vi "movimentacao_cin_inv_bezier.vi"() -> ()   [LabVIEW 2017]
doc: "The myRIO Project template acquires acceleration data from the onboard accelerometer and displays the changes of acceleration values in a waveform chart."
uses:
  <vilib>/Analysis/Matrix/Datatypes/RealMatrix.ctl
  <vilib>/myRIO/Instrument Drivers/Onboard IO/PWM/typedefs/PWM Reference.ctl
  <vilib>/myRIO/Common/Instrument Driver Framework/Utilities/typedefs/myRIO Generic Hardware Reference.ctl
  <vilib>/myRIO/Common/Instrument Driver Framework/Utilities/typedefs/Hardware Version Enum.ctl
  <vilib>/myRIO/Common/Instrument Driver Framework/Utilities/typedefs/myRIO v1.0 Reference.ctl
  <vilib>/myRIO/Common/Instrument Driver Framework/Utilities/typedefs/Generic FPGA Reference.ctl
  <vilib>/myRIO/Common/Instrument Driver Framework/myRIO v1.0/PWM/typedefs/PWM Channels Enum.ctl
  <vilib>/myRIO/Instrument Drivers/Onboard IO/PWM/typedefs/PWM Configuration.ctl
  <vilib>/userdefined/High Color/nirio_resource_hc.ctl
  <vilib>/myRIO/Common/Instrument Driver Framework/myRIO v1.0/PWM/vis/myRIO v1.1 Open PWM.vi
  <vilib>/myRIO/Common/Instrument Driver Framework/Utilities/vis/Validate Channels.vi
  <vilib>/myRIO/Common/Instrument Driver Framework/myRIO v1.0/PWM/vis/myRIO v1.0 Reserve PWM.vi
  <vilib>/myRIO/Instrument Drivers/Onboard IO/PWM/vis/Set Duty Cycle and Frequency.vi
  <vilib>/myRIO/Common/Instrument Driver Framework/myRIO v1.0/PWM/vis/myRIO v1.0 Close PWM.vi
  <vilib>/myRIO/Common/Instrument Driver Framework/myRIO v1.0/PWM/vis/myRIO v1.0 Build MUX Configuration PWM.vi
  <vilib>/myRIO/Common/Instrument Driver Framework/myRIO v1.0/Resource Manager/vis/myRIO v1.0 Reserve Channel List.vi
  <vilib>/myRIO/Common/Instrument Driver Framework/myRIO v1.0/PWM/vis/myRIO v1.0 Unreserve PWM.vi
  <vilib>/myRIO/Common/Instrument Driver Framework/myRIO v1.0/Resource Manager/vis/myRIO v1.0 Create Configuration List.vi
  <vilib>/myRIO/Common/Instrument Driver Framework/myRIO v1.0/Resource Manager/vis/myRIO v1.0 Reserve Channel.vi
  <vilib>/myRIO/Common/Instrument Driver Framework/myRIO v1.0/Resource Manager/vis/myRIO v1.0 Unreserve Channel.vi
  <vilib>/myRIO/Common/Instrument Driver Framework/myRIO v1.0/Resource Manager/vis/myRIO v1.0 Unreserve Channel List.vi
  <vilib>/myRIO/Common/Instrument Driver Framework/myRIO v1.0/Resource Manager/vis/myRIO v1.0 Build Mutex Name.vi
  <vilib>/Utility/VariantDataType/GetNumericInfo.vi
  <vilib>/Utility/error.llb/Error Cluster From Error Code.vi
  <vilib>/myRIO/Common/Instrument Driver Framework/myRIO v1.0/myRIO v1.1 Open.vi
  <vilib>/myRIO/Common/Instrument Driver Framework/Utilities/vis/IO Manager.vi
  <vilib>/myRIO/Common/Instrument Driver Framework/Utilities/vis/Configuration Manager.vi
  <vilib>/myRIO/Common/Instrument Driver Framework/myRIO v1.0/Resource Manager/vis/myRIO v1.0 Configure IO.vi
  <vilib>/myRIO/Common/Instrument Driver Framework/myRIO v1.0/myRIO v1.0 Close.vi
  <vilib>/myRIO/Common/Instrument Driver Framework/myRIO v1.0/PWM/vis/myRIO v1.0 Write PWM.vi
  <vilib>/myRIO/Common/Instrument Driver Framework/myRIO v1.0/PWM/vis/myRIO v1.0 Shutdown PWM.vi
  <vilib>/myRIO/Instrument Drivers/Onboard IO/PWM/vis/myRIO PWM Open.xnode
  <vilib>/myRIO/Instrument Drivers/Onboard IO/PWM/PWM.lvlib
  <vilib>/Analysis/Matrix/NI_Matrix.lvlib
panel:
  in  "String 3":string="(151,57;2,89;11,57);(245,79;-185,54;30);(126,28;-267,6;41,68);(43,16; -253,15;220,9);(-167,79;-132,49;100)"
  out "x .and. y?":bool
  in  "OK Button":bool
  out "subarray":dbl[](array[numeric])
  in  "String 2":string="(151,57;2,89;11,57);(245,79;-185,54;30);(126,28;-267,6;41,68);(43,16; -253,15;220,9);(-167,79;-132,49;100)"
  out "output array":T1
  out "appended array 2":dbl[](array[numeric])
  out "logical AND":bool
  out "x = y?":bool[](array[boolean])
  out "POS_E_ORIEN_HOME":dbl[](array[numeric])
  out "ANG_POSI_E_ORIEN_HOME":dbl[](array[numeric])
  out "CURRENT POSITIONS OF THE MOTORS":dbl[](array[numeric])
  in  "angulo_garra":dbl(knob) scale=-180.0..180.0
  in  "Duty Cycle Abert":dbl=0.04 format="%#_13g"
  out "Actuator 2":bool
  in  "Actuator":bool
  in  "Conveyor speed (mm/s)":dbl(slide)=200.0 step=1.0 scale=0.0..350.0
  out "indexador":i32
  out "Objeto detectado":bool
  out "Manipulando":bool
  out "Está em Home":bool
  out "Posicao_desejada":bool
  in  "Home":bool
  in  "error in (no error)":errorcluster
  in  "PARAR":bool
  in  "POSITION VECTOR":dbl[](array[numeric])
  # "ROTINA DE CONTROLE DO PROTÓTIPO DE FMS"
  # "COMANDO DE POSIÇÃO\nATUAL DOS MOTORES"
  # "OPERATION STATUS"
  # "ÂNGULOS DE JUNTAS"
  # "THETA 1"
  # "MOTOR 1"
  # "HOME"
  # "THETA 2"
  # "MOTOR 2"
  # "DESIRED POSITION"
  # "THETA 3"
  # "MOTOR 3"
  # "OBJECT DETECTED"
  # "THETA 4"
  # "MOTOR 4"
  # "MANIPULATING"
  # "THETA 5"
  # "MOTOR 5"
  # "ACTUATOR"
  # "MOTOR 6"
  # "VELOCIDADE DA ESTEIRA (mm/s)"
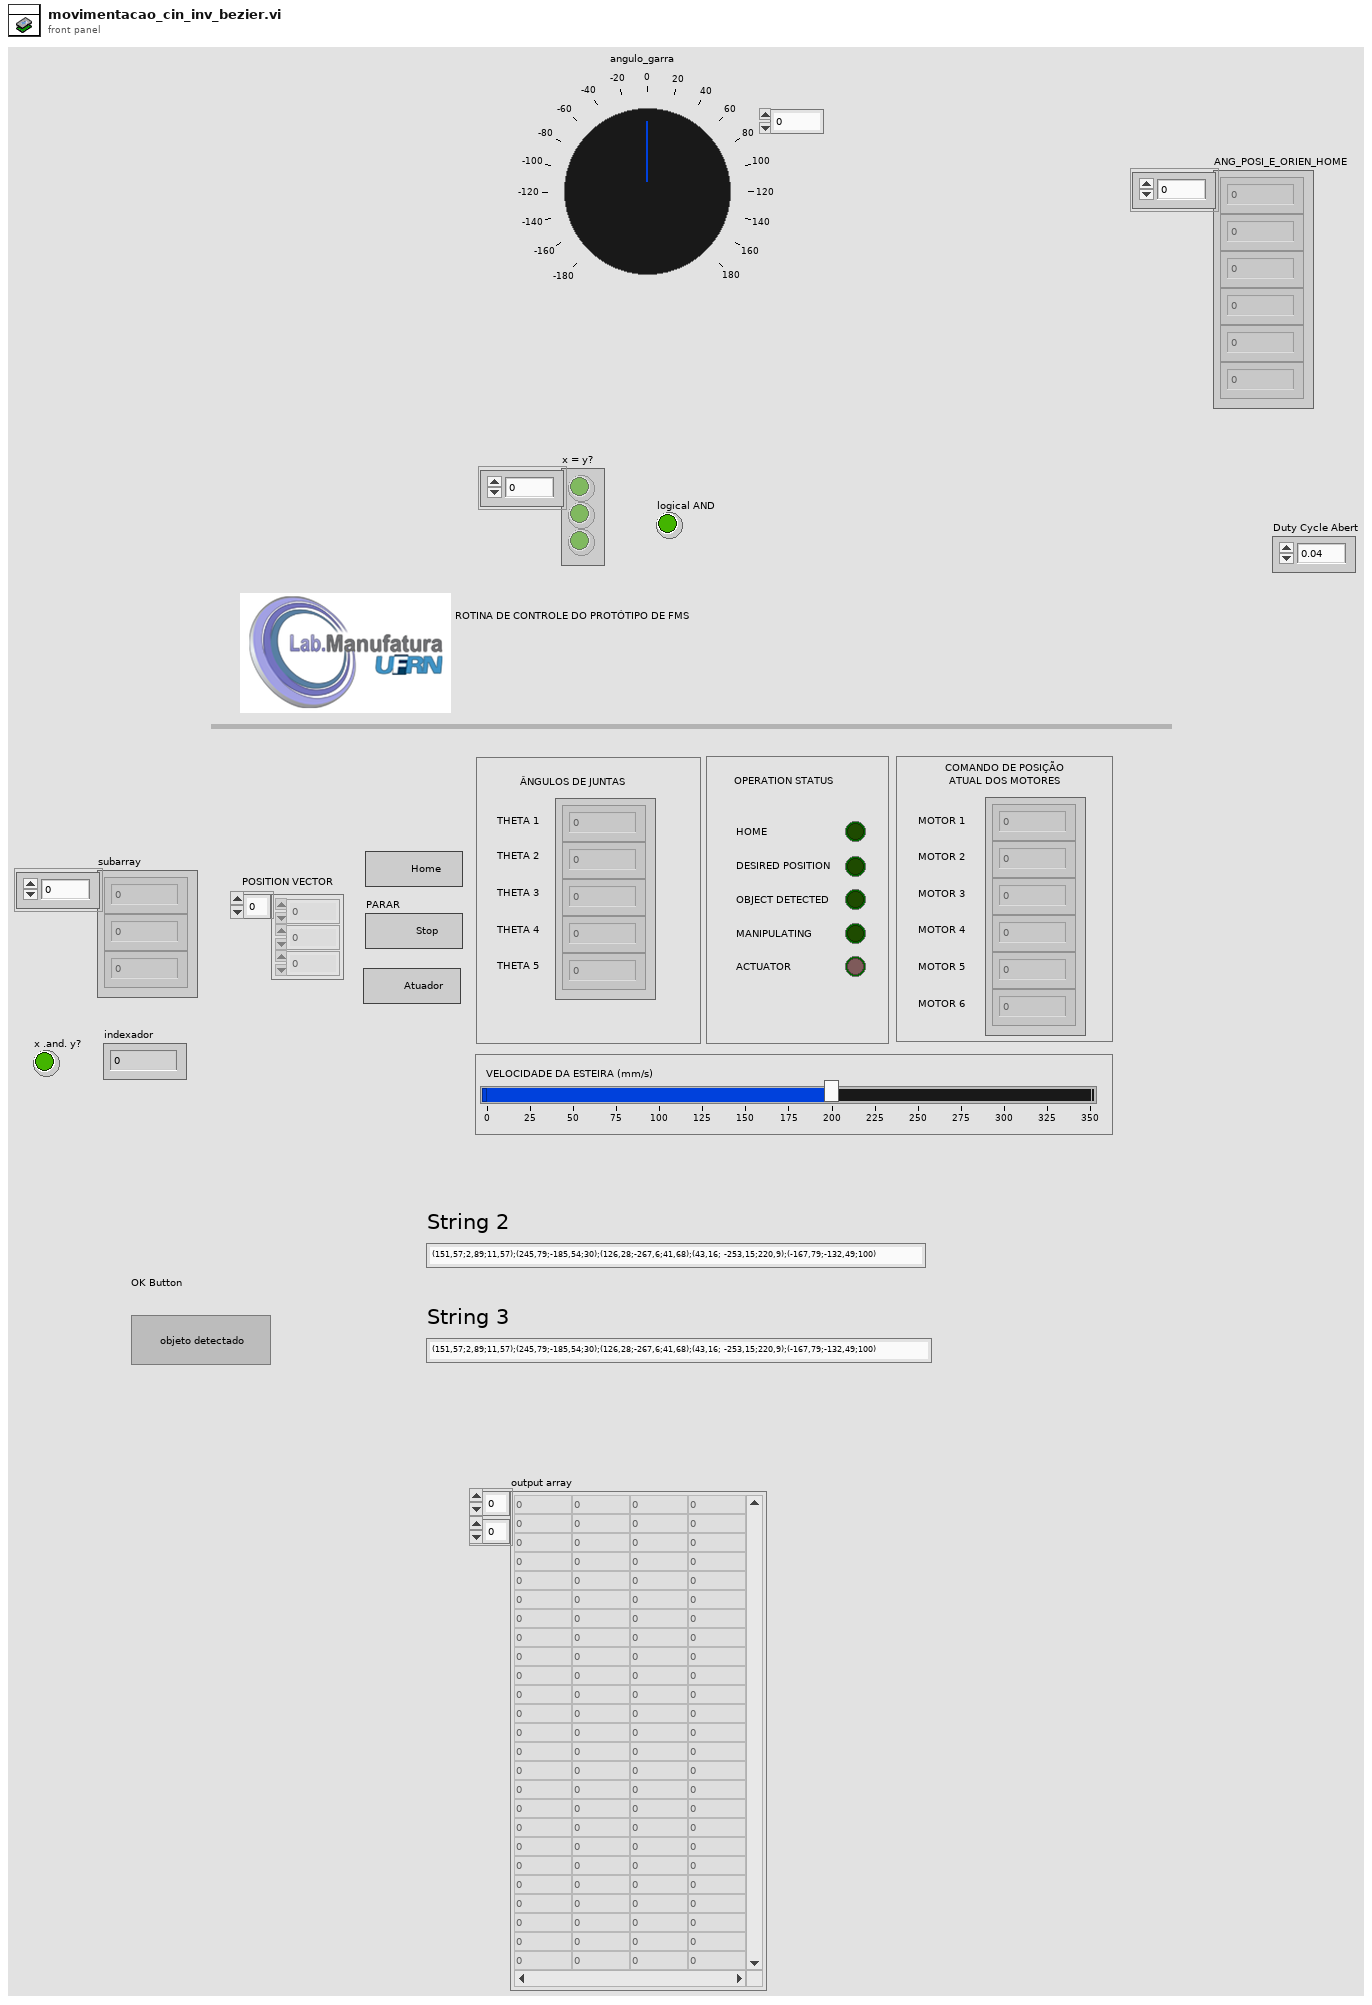
[diagram p1: front panel]
types:
  T1 = typedef "NI_Matrix.lvlib/RealMatrix.ctl" = dbl[][]
  T2 = cluster{"theta 1":dbl, "theta 2":dbl, "theta 3":dbl, "theta5":dbl, "theta4":dbl}
  T3 = typedef "nirio_resource_hc.ctl" = tag
  T4 = typedef "Hardware Version Enum.ctl" = enum16{"Unknown", "myRIO-1900", "myRIO-1950", "roboRIO", "NI ELVIS RIO CM"}
  T5 = typedef "PWM.lvlib/PWM Reference.ctl" = cluster{"myRIO Reference":T6, "PWM Channels Enum":T9, "PWM Configuration":T10}
  T6 = typedef "myRIO Generic Hardware Reference.ctl" = cluster{"myRIO Model":T4, "myRIO Hardware Reference":T7}
  T7 = typedef "myRIO v1.0 Reference.ctl" = cluster{"Generic FPGA Reference":T8, "Allow multiple opens":bool}
  T8 = typedef "Generic FPGA Reference.ctl" = refnum<k20>
  T9 = typedef "PWM Channels Enum.ctl" = enum16{"Not Connected", "C/PWM0", "C/PWM1", "A/PWM0", "A/PWM1", "A/PWM2", "B/PWM0", "B/PWM1", "B/PWM2", "PWM/PWM0", "PWM/PWM1", "PWM/PWM2", "PWM/PWM3", "PWM/PWM4", "PWM/PWM5", "PWM/PWM6", "PWM/PWM7", "PWM/PWM8", "PWM/PWM9"}
  T10 = typedef "PWM.lvlib/PWM Configuration.ctl" = cluster{"Frequency":dbl, "Duty Cycle":dbl}
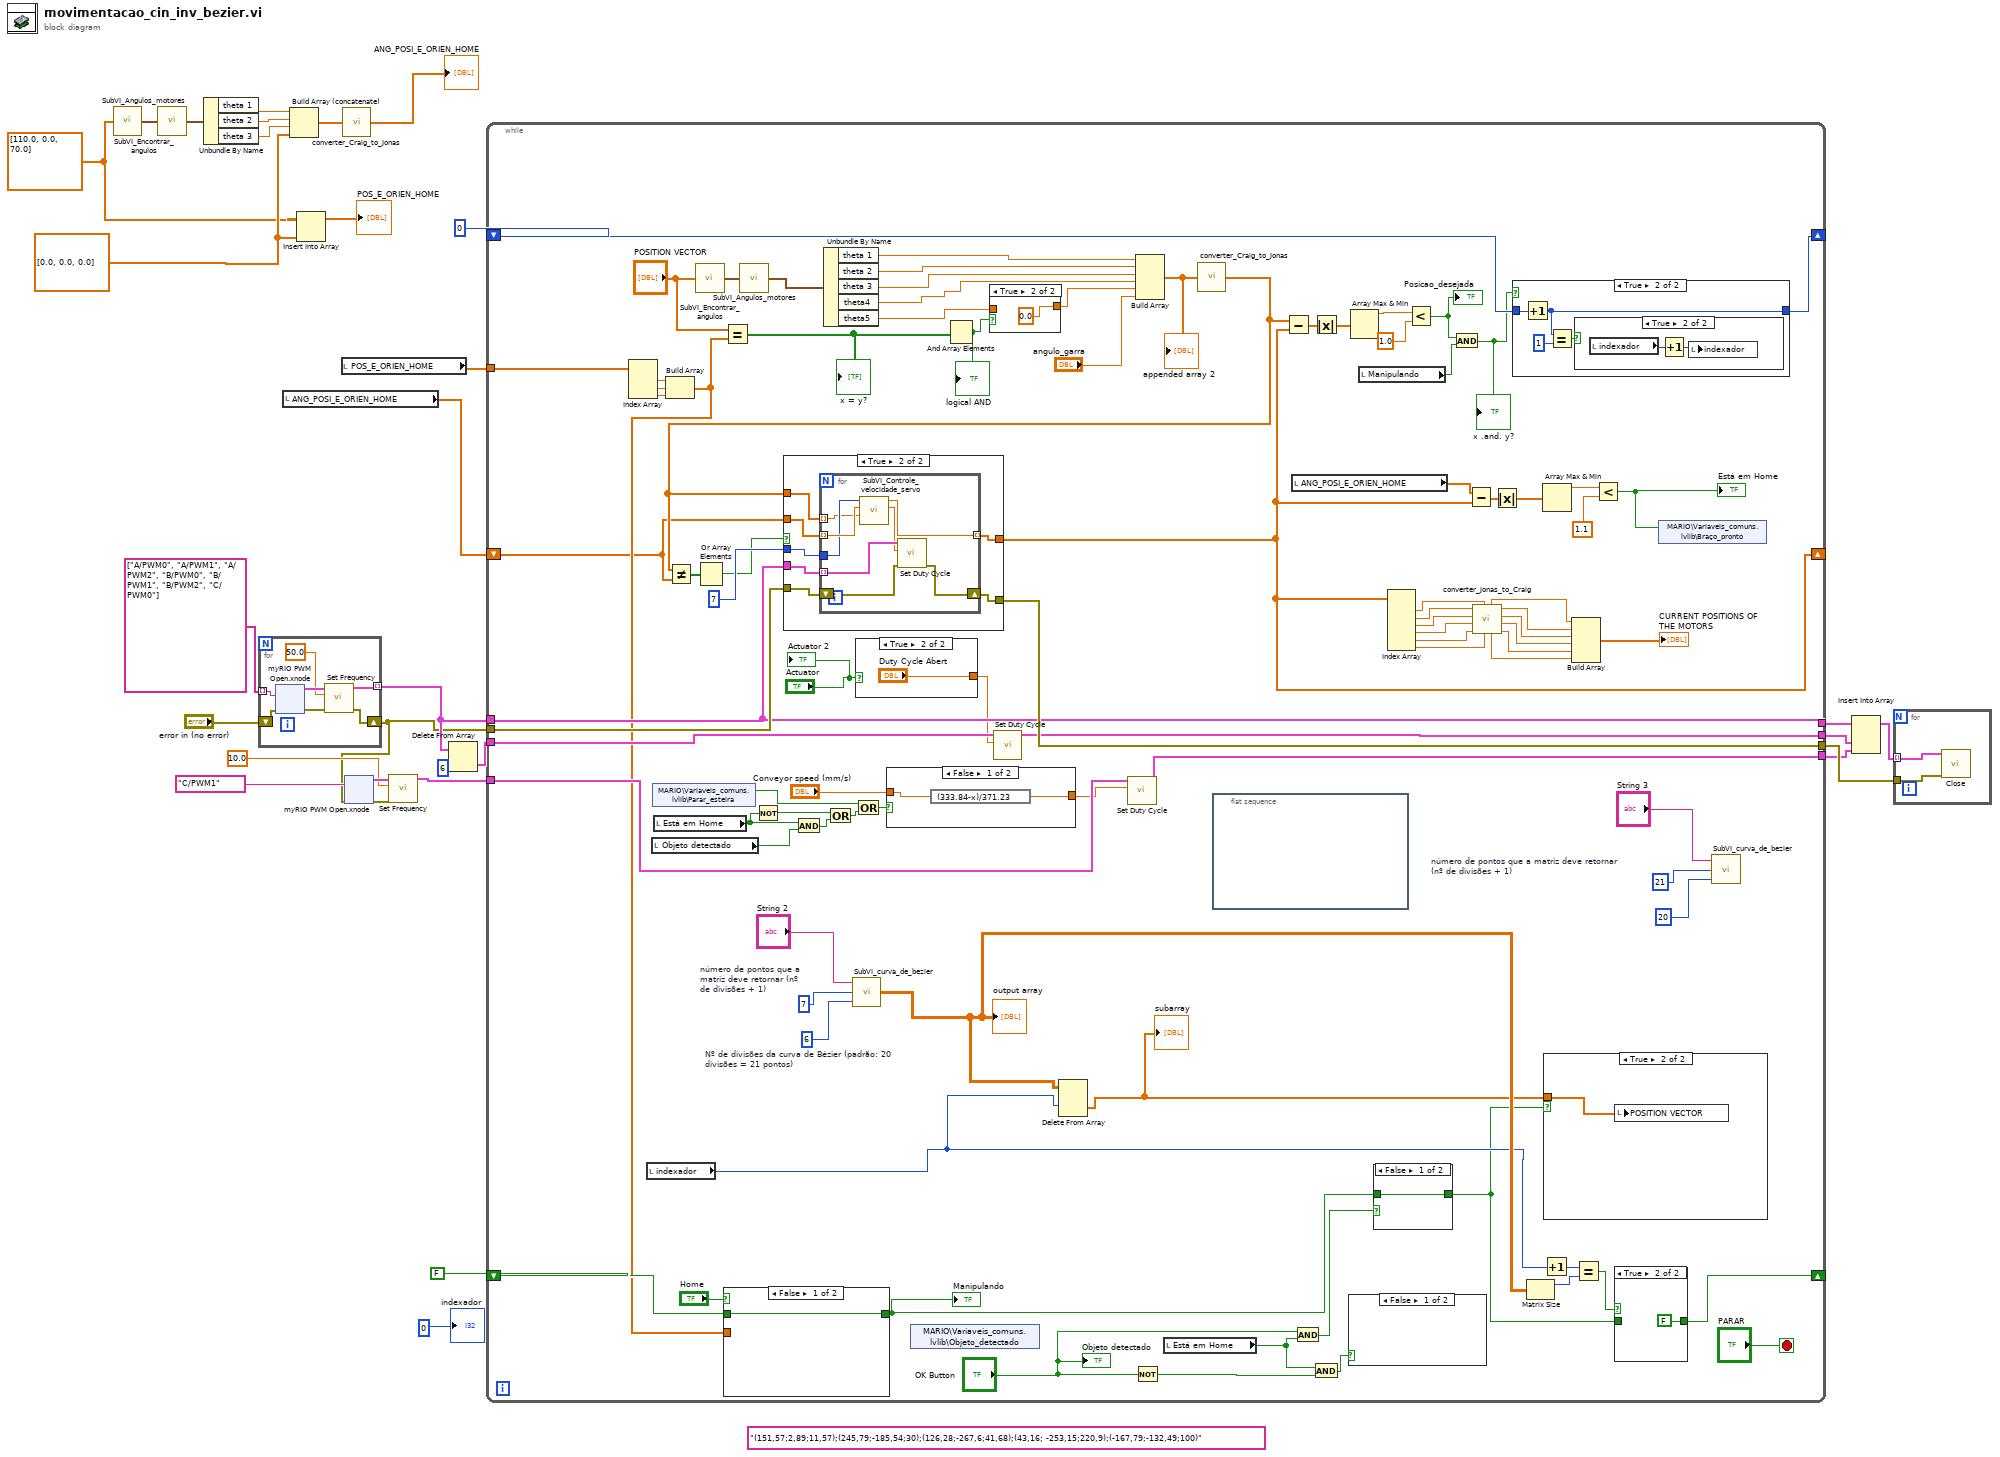
[diagram p0: block diagram]
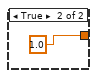
[diagram p3: hidden frame]
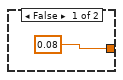
[diagram p4: hidden frame]
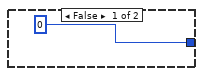
[diagram p7: hidden frame]
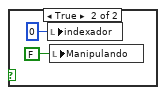
[diagram p9: hidden frame]
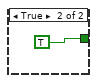
[diagram p10: hidden frame]
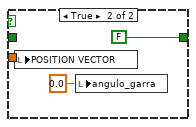
[diagram p11: hidden frame]
diagram:
  (unwired) "(151,57;2,89;11,57);(245,79;-185,54;30);(126,28;-267,6;41,68);(43,16; -253,15;220,9);(-167,79;-132,49;100)" ("String 2")
  w8 = dbl[] [0.0, 0.0, 0.0] ("vetor_P")
  w3 = dbl[] [110.0, 0.0, 70.0] ("vetor_P")
  n1 = call "SubVI_Encontrar_angulos.vi"("vetor_P"=w3) -> ("ângulos de Juntas"=w2:T2)
  n2 = call "SubVI_Angulos_motores.vi"("input cluster"=w2) -> ("output cluster"=w1:T2)
  n3 = Unbundle By Name(w1) -> ("theta 1"=w12:dbl, "theta 2"=w11:dbl, "theta 3"=w10:dbl)
  n4 = for {
    tunnel: tag[] ["A/PWM0", "A/PWM1", "A/PWM2", "B/PWM0", "B/PWM1", "B/PWM2", "C/PWM0"] -> [w35] mode=indexing
    tunnel: [w34] -> w25 mode=indexing
    shift-right: [w33] -> w14
    shift-left: "error in (no error)" -> [w32]
    n5 = xnode ("myRIO PWM Open.xnode")("error in (no error)"=w32, "Channel Name"=w35) -> ("error out"=w36:errorcluster, "PWM Ref Out"=w38:T5)  [unwired: 1 in]
    n6 = call <vilib>:"Set Frequency.vi"("error in (no error)"=w36, "Frequency [Hz]"=50.0, "PWM Ref In"=w38) -> ("error out"=w33:errorcluster, "PWM Ref Out"=w34:T5)  [unwired: 6 in]
  }
  n7 = local read "ANG_POSI_E_ORIEN_HOME"() -> (w9:dbl[])
  n8 = Build Array (concatenate)(w12, w11, w10, w8) -> (w5:dbl[])
  n9 = Insert Into Array(array=w3, new element=w8) -> (→"POS_E_ORIEN_HOME":dbl[])  [unwired: 1 in]
  n10 = local read "POS_E_ORIEN_HOME"() -> (w6:dbl[])
  n11 = call "converter_Craig_to_Jonas.vi"("array"=w5) -> ("appended array"=→"ANG_POSI_E_ORIEN_HOME":dbl[])
  n12 = xnode "myRIO PWM Open.xnode"("error in (no error)"=w14, "Channel Name"=tag "C/PWM1") -> ("error out"=w18:errorcluster, "PWM Ref Out"=w19:T5)  [unwired: 1 in]
  n13 = call <vilib>:"Set Frequency.vi"("error in (no error)"=w18, "Frequency [Hz]"=10.0, "PWM Ref In"=w19) -> ("PWM Ref Out"=w15:T5)  [unwired: 6 in, 1 out]
  n14 = Delete From Array(array=w25, index=6) -> (deleted portion=w23:T5)  [unwired: 1 in, 1 out]
  n15 = while {
    tunnel: [w146] -> w31
    shift-right: [w76] -> _
    shift-left: w9 -> [w68]
    tunnel: w14 -> [w144]
    tunnel: w25 -> [w143]
    tunnel: [w143] -> w22
    shift-right: [w60] -> _
    shift-left: FALSE -> [w126]
    shift-right: [w135] -> _
    shift-left: u32 0 ("ms to wait (braço)") -> [w134]
    tunnel: w23 -> [w121]
    tunnel: [w120] -> w21
    tunnel: w15 -> [w118]
    tunnel: [w114] -> w13
    tunnel: w6 -> [w84]
    stop <- "PARAR" stop-if-true
    w56 = i64 21  # número de pontos que a matriz deve retornar (nº de divisões + 1)
    w58 = 6  # Nº de divisões da curva de Bézier (padrão: 20 divisões = 21 pontos)
    w66 = i64 7  # número de pontos que a matriz deve retornar (nº de divisões + 1)
    n16 = Index Array(array=w84) -> (element #1=w87:dbl, element #2=w86:dbl, element #3=w85:dbl)  [unwired: 3 in]
    n17 = local read "indexador"() -> (w63:i32)
    n18 = local read "Objeto detectado"() -> (w111:bool)
    n19 = shared-variable "MARIO\\Variaveis_comuns.lvlib\\Parar_esteira"() -> (w113:bool)  [unwired: 1 in, 1 out]
    n20 = local read "Está em Home"() -> (w108:bool)
    n21 = Build Array(w87, w86, w85) -> (w83:dbl[])
    n22 = call "SubVI_Encontrar_angulos.vi"("vetor_P"="POSITION VECTOR") -> ("ângulos de Juntas"=w73:T2)
    n23 = Equal?(x="POSITION VECTOR", y=w83) -> (x = y?=w124:bool[])
    "x = y?" <- w124
    n24 = case shown="False" "Home" {
      tunnel: w83 -> [_ w172]
      tunnel: w126 -> [w169 _]
      tunnel: [w169 FALSE ("Manipulando")] -> w75
      frame False {
      }
      frame True {
        n25 = local write "POSITION VECTOR"(w172) -> ()
        n26 = local write "angulo_garra"(0.0 ("angulo_garra")) -> ()
      }
    }
    "Manipulando" <- w75
    n27 = call "SubVI_Angulos_motores.vi"("input cluster"=w73) -> ("output cluster"=w72:T2)
    n28 = Not(x=w108) -> (.not. x?=w109:bool)
    n29 = And(x=w108, y=w111) -> (x .and. y?=w110:bool)
    n30 = Unbundle By Name(w72) -> ("theta 1"=w93:dbl, "theta 2"=w92:dbl, "theta 3"=w91:dbl, "theta4"=w71:dbl, "theta5"=w70:dbl)
    n31 = Or(x=w109, y=w110) -> (x .or. y?=w107:bool)
    n32 = call "SubVI_curva_de_bezier.vi"("Nº de divisões da curva de Bézier (padrão: 20 divisões = 21 pontos)"=w58, "número de pontos que a matriz deve retornar (padrão: nº de divisões + 1)"=w66, "String in"="String 2") -> ("matrix"=w65:T1)
    "output array" <- w65
    n33 = Or(x=w113, y=w107) -> (x .or. y?=w115:bool)
    n34 = case shown="True" "Actuator" {
      tunnel: [0.08 ("Duty Cycle Abert") "Duty Cycle Abert"] -> w119
      frame False {
      }
      frame True {
      }
    }
    n35 = case shown="False" w115 {
      tunnel: [w150 1.0 ("Duty Cycle")] -> w117
      tunnel: "Conveyor speed (mm/s)" -> [w149 _]
      frame False {
        n36 = expression code="(333.84-x)/371.23"(w149) -> (w150:dbl)
      }
      frame True {
      }
    }
    n37 = shared-variable "MARIO\\Variaveis_comuns.lvlib\\Objeto_detectado"() -> ()  [unwired: 1 in, 2 out]
    n38 = And Array Elements(Boolean array=w124) -> (logical AND=w123:bool)
    "logical AND" <- w123
    n39 = case shown="True" w123 {
      tunnel: [w154 0.0 ("theta5")] -> w90
      tunnel: w70 -> [w154 _]
      frame False {
      }
      frame True {
      }
    }
    n40 = call <vilib>:"Set Duty Cycle.vi"("Duty Cycle"=w119, "PWM Ref In"=w121) -> ("PWM Ref Out"=w120:T5)  [unwired: 7 in, 1 out]
    n41 = Delete From Array(array=w65, index (row)=w63) -> (deleted portion=w62:dbl[])  [unwired: 2 in, 1 out]
    "subarray" <- w62
    n42 = call <vilib>:"Set Duty Cycle.vi"("Duty Cycle"=w117, "PWM Ref In"=w118) -> ("PWM Ref Out"=w114:T5)  [unwired: 7 in, 1 out]
    n43 = Not(x="OK Button") -> (.not. x?=w79:bool)
    n44 = Build Array(w93, w92, w91, w71, w90, "angulo_garra") -> (w89:dbl[])
    "appended array 2" <- w89
    n45 = local read "Está em Home"() -> (w80:bool)
    n46 = call "converter_Craig_to_Jonas.vi"("array"=w89) -> ("appended array"=w82:dbl[])
    n47 = Not Equal?(x=w82, y=w68) -> (x != y?=w142:bool[])
    n48 = Or Array Elements(Boolean array=w142) -> (logical OR=w141:bool)
    n49 = case shown="True" w141 {
      tunnel: [w173 w181] -> w146
      tunnel: w144 -> [w173 w180]
      tunnel: w143 -> [_ w179]
      tunnel: w68 -> [w174 w178]
      tunnel: [w174 w176] -> w76
      tunnel: u32 7 ("ms to wait (braço)") -> [_ w177]
      tunnel: w82 -> [_ w175]
      frame False {
      }
      frame True {
        n50 = for {
          tunnel: w179 -> [w187] mode=indexing
          tunnel: w178 -> [w186] mode=indexing
          tunnel: w177 -> [w184]
          tunnel: [w183] -> w176 mode=indexing
          tunnel: w175 -> [w182] mode=indexing
          shift-right: [w189] -> w181
          shift-left: w180 -> [w188]
          n51 = call "SubVI_Controle_velocidade_servo.vi"("Posição Desejada"=w182, "Posição"=w186, "milliseconds to wait"=w184) -> ("Duty Cycle"=w185:dbl, "Posição"=w183:dbl)  [unwired: 7 in]
          n52 = call <vilib>:"Set Duty Cycle.vi"("error in (no error)"=w188, "Duty Cycle"=w185, "PWM Ref In"=w187) -> ("error out"=w189:errorcluster)  [unwired: 6 in, 1 out]
        }
      }
    }
    n53 = flat-sequence {
      frame #0 {
      }
    }
    n54 = Subtract(x=w82, y=w76) -> (x-y=w140:dbl[])
    n55 = local read "ANG_POSI_E_ORIEN_HOME"() -> (w88:dbl[])
    n56 = And(x="OK Button", y=w80) -> (x .and. y?=w137:bool)
    n57 = Absolute Value(x=w140) -> (abs(x)=w139:dbl[])
    n58 = And(x=w80, y=w79) -> (x .and. y?=w131:bool)
    n59 = case shown="False" w131 {
      frame False {
      }
      frame True {
        n60 = local write "indexador"(0 ("indexador")) -> ()
        n61 = local write "Manipulando"(FALSE ("Manipulando")) -> ()
      }
    }
    n62 = Array Max & Min(array=w139) -> (max value=w81:dbl)  [unwired: 3 out]
    n63 = local read "Manipulando"() -> (w133:bool)
    n64 = case shown="False" w137 {
      tunnel: [w167 TRUE] -> w61
      tunnel: w75 -> [w167 _]
      frame False {
      }
      frame True {
      }
    }
    n65 = Index Array(array=w76) -> (element #1=w106:dbl, element #2=w105:dbl, element #3=w104:dbl, element #4=w103:dbl, element #5=w102:dbl, element #6=w101:dbl)  [unwired: 6 in]
    n66 = Less?(x=w81, y=1.0) -> (x < y?=w77:bool)
    "Posicao_desejada" <- w77
    n67 = And(x=w77, y=w133) -> (x .and. y?=w132:bool)
    "x .and. y?" <- w132
    n68 = Subtract(x=w88, y=w76) -> (x-y=w130:dbl[])
    n69 = call "converter_Jonas_to_Craig.vi"("theta6Jonas"=w101, "theta1Jonas"=w106, "theta5Jonas"=w102, "theta4Jonas"=w103, "theta3Jonas"=w104, "theta2Jonas"=w105) -> ("theta5Craig"=w96:dbl, "theta4Craig"=w97:dbl, "theta3Craig"=w98:dbl, "theta2Craig"=w99:dbl, "theta6Craig"=w95:dbl, "theta1Craig"=w100:dbl)
    n70 = Absolute Value(x=w130) -> (abs(x)=w129:dbl[])
    n71 = case shown="True" w132 {
      tunnel: w134 -> [_ w162]
      tunnel: [u32 0 ("ms to wait (braço)") w161] -> w135
      frame False {
      }
      frame True {
        n72 = Increment(x=w162) -> (x+1=w161:u32)
        n73 = Equal?(x=w161, y=u32 1) -> (x = y?=w159:bool)
        n74 = case shown="True" w159 {
          frame False {
          }
          frame True {
            n75 = local read "indexador"() -> (w164:i32)
            n76 = Increment(x=w164) -> (x+1=w163:i32)
            n77 = local write "indexador"(w163) -> ()
          }
        }
      }
    }
    n78 = Matrix Size(0:w65) -> (1:w59:i32)  [unwired: 1 out]
    n79 = Increment(x=w63) -> (x+1=w78:i32)
    n80 = Array Max & Min(array=w129) -> (max value=w128:dbl)  [unwired: 3 out]
    n81 = case shown="True" w61 {
      tunnel: w62 -> [_ w148]
      frame False {
      }
      frame True {
        n82 = local write "POSITION VECTOR"(w148) -> ()
      }
    }
    n83 = Build Array(w100, w99, w98, w97, w96, w95) -> (→"CURRENT POSITIONS OF THE MOTORS":dbl[])
    n84 = Equal?(x=w78, y=w59) -> (x = y?=w125:bool)
    n85 = Less?(x=w128, y=1.1) -> (x < y?=w112:bool)
    "Está em Home" <- w112
    n86 = case shown="True" w125 {
      tunnel: [w156 FALSE ("Manipulando")] -> w60
      tunnel: w61 -> [w156 _]
      frame False {
      }
      frame True {
      }
    }
    n87 = shared-variable "MARIO\\Variaveis_comuns.lvlib\\Braço_pronto"(w112) -> ()  [unwired: 1 in, 1 out]
    n88 = call "SubVI_curva_de_bezier.vi"("Nº de divisões da curva de Bézier (padrão: 20 divisões = 21 pontos)"=20, "número de pontos que a matriz deve retornar (padrão: nº de divisões + 1)"=w56, "String in"="String 3") -> ()  [unwired: 1 out]
    "Objeto detectado" <- "OK Button"
    "Actuator 2" <- "Actuator"
  }
  n89 = Insert Into Array(array=w22, new element #1=w21, new element #2=w13) -> (w20:T5[])  [unwired: 1 in]
  n90 = for {
    tunnel: w31 -> [w191]
    tunnel: w20 -> [w190] mode=indexing
    n91 = call <vilib>:"Close.vi"("error in (no error)"=w191, "PWM Ref In"=w190) -> ()  [unwired: 9 in, 1 out]
  }
  "indexador" <- 0
